vi "CardChannel2MuxChannel.vi"(7 "Probe Card Channels":i32=32, 8 "error in (no error)":errorcluster, 10 "Probecard Channel No.":i32=1 min=1 max=26 step=1, 11 "LXIPXISwitching in":refnum<class "LXIPXISwitching.lvclass">) -> (0 "error out":errorcluster, 1 "Bank":i32=1 min=1 max=2 step=1, 2 "Mux No.:":u32(ring)=1 items=["", "", "", "", "MUX1", "MUX2"], 3 "LXIPXISwitching out":refnum<class "LXIPXISwitching.lvclass">, 4 "Channel":i32=1 min=1 max=8 step=1, 5 "Mux No. string":string)   [LabVIEW 2019, in "LXIPXISwitching.lvclass"]
doc: "For striptests: translate probecard channel number to MUX channel"
uses:
  LXIPXISwitching.lvclass
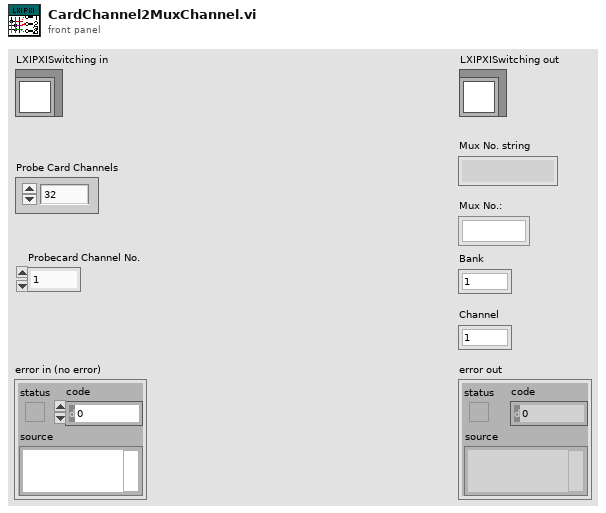
[diagram p1: front panel]
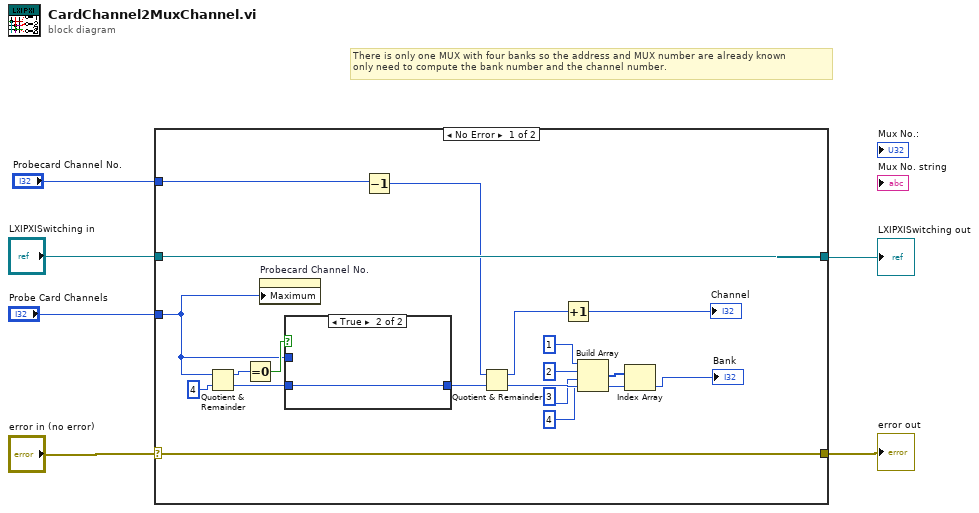
[diagram p0: block diagram]
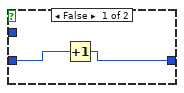
[diagram p2: hidden frame]
diagram:
  # "There is only one MUX with four banks so the address and MUX number are already known\nonly need to compute the bank number and the channel number."
  n1 = case shown="No Error" "error in (no error)" {
    selector: "error in (no error)" -> [w25 w29]
    tunnel: [w25 w29] -> w5
    tunnel: [w24 w30] -> w3
    tunnel: "LXIPXISwitching in" -> [w24 w30]
    tunnel: "Probe Card Channels" -> [w13 _]
    tunnel: "Probecard Channel No." -> [w8 _]
    frame No Error {
      n2 = Quotient & Remainder(x=w13, y=4) -> (x-y*floor(x/y)=w17:i32, floor(x/y)=w18:i32)
      n3 = Equal To 0?(x=w17) -> (x = 0?=w16:bool)
      n4 = property on="Probecard Channel No." class="DigNum (strict)"("Maximum"=w13) -> ()  [unwired: 2 in, 2 out]
      n5 = case shown="True" w16 {
        tunnel: w13 -> [_ _]
        tunnel: w18 -> [w27 w28]
        tunnel: [w26 w28] -> w19
        frame False {
          n6 = Increment(x=w27) -> (x+1=w26:i32)
        }
        frame True {
        }
      }
      n7 = Decrement(x=w8) -> (x-1=w7:i32)
      n8 = Quotient & Remainder(x=w7, y=w19) -> (x-y*floor(x/y)=w15:i32, floor(x/y)=w23:i32)
      n9 = Increment(x=w15) -> (x+1=→"Channel":i32)
      n10 = Build Array(1, 2, 3 ("element"), 4 ("element")) -> (w22:i32[])
      n11 = Index Array(array=w22, index=w23) -> (element=→"Bank":i32)
    }
    frame Error {
    }
  }
  "error out" <- w5
  "LXIPXISwitching out" <- w3
